vi "Laboratory_practice1.vi"() -> ()   [LabVIEW 2022 SP3]
panel:
  out "km/h":dbl
  in  "m/s":dbl
  out "km/h":dbl(knob) scale=0.0..100.0
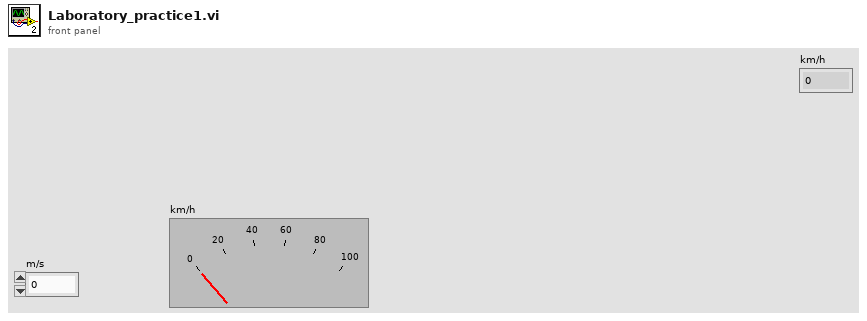
[diagram p1: front panel]
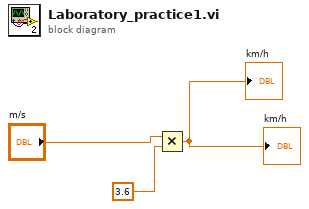
[diagram p0: block diagram]
diagram:
  n1 = Multiply(x="m/s", y=3.6 ("x")) -> (x*y=→"km/h" →"km/h":dbl)
